vi "Words To Network-Order Bytes I8.vi"(1 "word":i8 format="%02x") -> (0 "bytes":u8[](array[numeric]) format="%02x")   [LabVIEW 2020, in "NI_Bit Manipulation.lvlib"]
uses:
  <vilib>/Bit Manipulation/NI_Bit Manipulation.lvlib
  3451642c-1dfe-4f1f-97de-8771b4fa65f6.vi
  3451642c-1dfe-4f1f-97de-8771b4fa65f6.vi/c9ade28e-b385-3fe8-d538-dffd9d47ee3f.vi
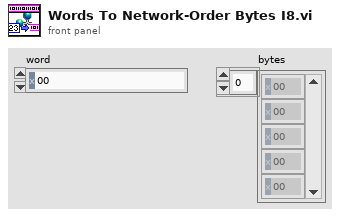
[diagram p1: front panel]
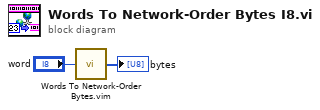
[diagram p0: block diagram]
diagram:
  n1 = call "Words To Network-Order Bytes.vim"("word"="word") -> ("bytes"=→"bytes":i8[])
